vi "String_send.vi"(8 "连接ID":refnum<k5>, 10 "data":string="hello", 11 "topic":string="/chatter") -> (0 "连接ID输出":refnum<k5>, 3 "JSON":string)   [LabVIEW 2014]
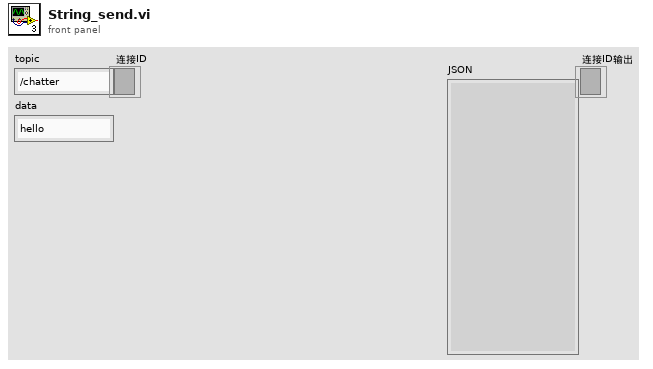
[diagram p1: front panel]
types:
  T1 = cluster{"op":string, "topic":string, "msg":cluster{"data":string}}
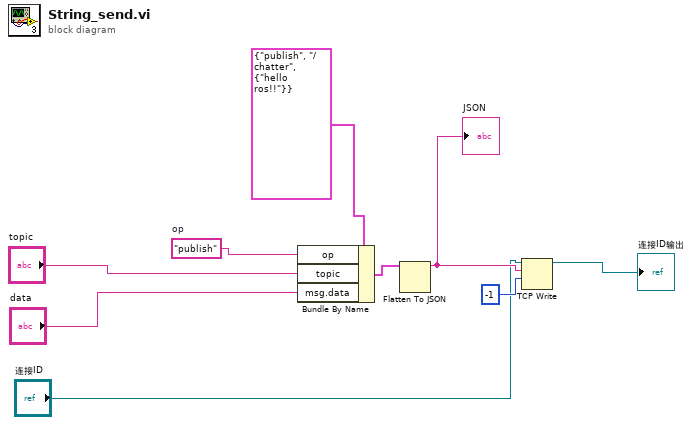
[diagram p0: block diagram]
diagram:
  w8 = "publish"  # op
  n1 = Bundle By Name(cluster=T1 {"op"="publish", "topic"="/chatter", "msg"={"data"="hello ros!!"}}, "op"=w8, "topic"="topic", "msg.data"="data") -> (w5:T1)
  n2 = Flatten To JSON(anything=w5) -> (JSON string=w3:string)  [unwired: 2 in, 1 out]
  "JSON" <- w3
  n3 = TCP Write(connection ID="连接ID", data in=w3, 9:-1 ("超时毫秒(25000)")) -> (connection ID out=→"连接ID输出":refnum<k5>)  [unwired: 1 in, 2 out]
